vi "Set Initialize Edit Sensor.vi"(8 "error in (no error)":errorcluster, 10 "Initialize Edit Sensor":bool, 11 "Abstract Initialize Edit Sensor Msg in":refnum<class "Abstract Initialize Edit Sensor Msg.lvclass">) -> (0 "error out":errorcluster, 3 "Abstract Initialize Edit Sensor Msg out":refnum<class "Abstract Initialize Edit Sensor Msg.lvclass">)   [LabVIEW 2013, in "Edit Sensor Model.lvlib" / "Abstract Initialize Edit Sensor Msg.lvclass"]
uses:
  Abstract Initialize Edit Sensor Msg.lvclass
  Abstract Initialize Edit Sensor Msg.lvclass/Abstract Initialize Edit Sensor Msg.ctl
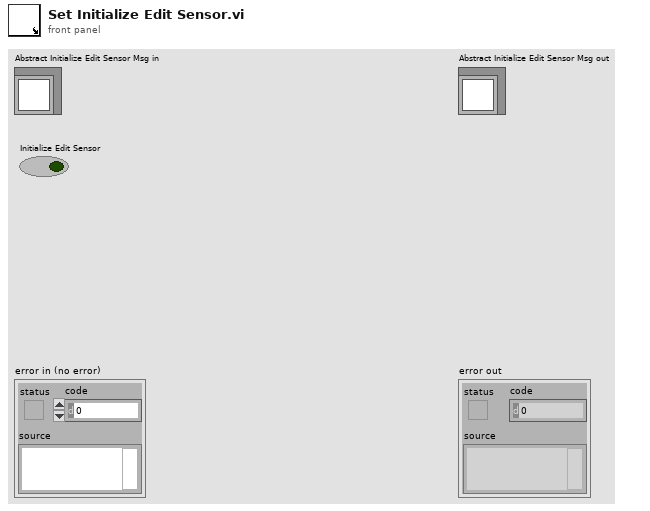
[diagram p1: front panel]
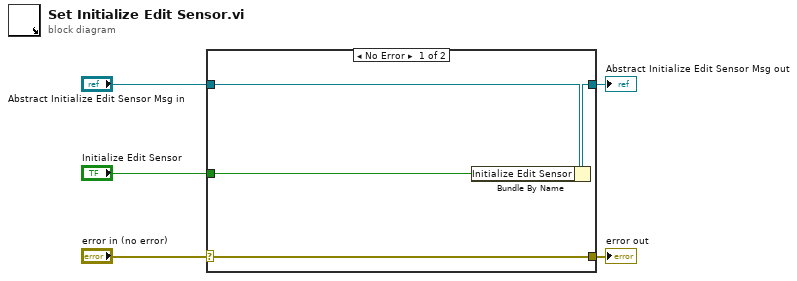
[diagram p0: block diagram]
diagram:
  n1 = case shown="No Error" "error in (no error)" {
    selector: "error in (no error)" -> [w9 w10]
    tunnel: [w9 w10] -> w4
    tunnel: [w7 w11] -> w2
    tunnel: "Abstract Initialize Edit Sensor Msg in" -> [w8 w11]
    tunnel: "Initialize Edit Sensor" -> [w6 _]
    frame No Error {
      n2 = Bundle By Name(cluster=w8, "Initialize Edit Sensor"=w6) -> (w7:refnum<class "Abstract Initialize Edit Sensor Msg.lvclass">)
    }
    frame Error {
    }
  }
  "error out" <- w4
  "Abstract Initialize Edit Sensor Msg out" <- w2
